vi "Quick Scale.vi"   [LabVIEW 2017, in "NI_AALBase.lvlib"]
doc: "Determines the maximum absolute value of the input <B>X</B> and then scales <B>X</B> using this value."
uses:
  NI_AALBase.lvlib
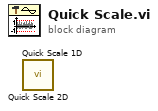
[diagram p0: block diagram]
diagram:
  n1 = call "Quick Scale 2D.vi"() -> ()  [unwired: 1 in, 3 out]
  n2 = call "Quick Scale 1D.vi"() -> ()  [unwired: 1 in, 3 out]
